vi "CALC_MARK_FUNC_DOM_USER.vi"(0 "VISA IN":refnum<visa-resource-name>, 1 "Marker number":i32, 2 "Range":i32, 5 "error in":errorcluster, 7 "Channel":i32) -> (14 "VISA Out":refnum<visa-resource-name>, 19 "error out":errorcluster)   [LabVIEW 2018, in "PNA-X.lvlib"]
doc: "CALCulate<cnum>:MARKer<mkr>:FUNCtion:DOMain:USER <range> \n(Read-Write) Assigns the specified marker to a range number. The x-axis travel of the marker is \nconstrained to the range's span. The span is specified with the \nCALC:MARK:FUNC:DOM:USER:START and STOP commands, unless range 0 is specified which \nis the full span of the analyzer. \nEach channel has 16 user ranges. (Trace statistics use the same ranges.) More than one marker can use \na domain range. \nSee Critical Note \nParameters \n<cnum> Channel number of the measurement. There must be a selected measurement \non that channel. If unspecified, <cnum> is set to 1. \n<mkr> Any marker number from 1 to 10; if unspecified, value is set to 1 \n<span> User span. Choose any Integer from 0 to 16 \n0 is Full Span of the analyzer \n1 to 16 are available for user-defined x-axis span \nExamples CALC:MARK:FUNC:DOM:USER 1 \ncalculate2:marker8:function:domain:user 1 \nQuery Syntax CALCulate<cnum>:MARKer<mkr>:FUNCtion:DOMain:USER? \nReturns the user span number that the specified marker is assigned to. \nReturn Type Numeric \nDefault 0 - Full Span"
uses:
  PNA-X.lvlib
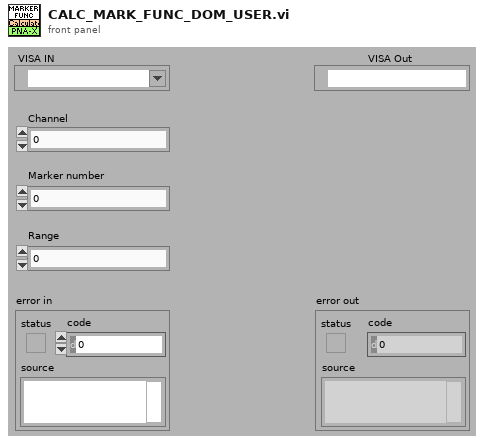
[diagram p1: front panel]
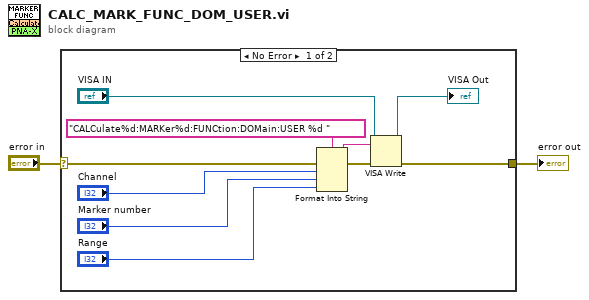
[diagram p0: block diagram]
diagram:
  n1 = case shown="No Error" "error in" {
    selector: "error in" -> [w12 w13]
    tunnel: [w7 w13] -> w1
    frame No Error {
      n2 = Format Into String(format string="CALCulate%d:MARKer%d:FUNCtion:DOMain:USER %d " ("Cmdline"), error in=w12, "Channel", "Marker number", "Range") -> (resulting string=w10:string, error out=w11:errorcluster)  [unwired: 1 in]
      n3 = VISA Write(VISA resource name="VISA IN", write buffer=w10, error in (no error)=w11) -> (VISA resource name out=→"VISA Out":refnum<visa-resource-name>, error out=w7:errorcluster)  [unwired: 1 out]
    }
    frame Error {
    }
  }
  "error out" <- w1
